vi "Get Public Events.vi"(8 "error in (no error)":errorcluster, 11 "LogEngine.lvclass":refnum<class "LogEngine.lvclass">) -> (0 "error out":errorcluster, 2 "PublicEvents":T1, 3 "LogEngine.lvclass":refnum<class "LogEngine.lvclass">)   [LabVIEW 2017, in "LogEngine.lvclass"]
doc: "Developed by Kevin Thompson\nkevin@thompsonengineering.net\n\nCopyright 2018-2020\nThompson Engineering, LLC"
uses:
  LogEngine.lvclass
  Data Types/TD LogEngine PublicEvents--cluster.ctl
  Ichor_Common/DataTypes/TD Async CmdMsg EventData--cluster.ctl
  Data Types/TD LoggerStateChanged EventData--cluster.ctl
  Data Types/TD Logger State Data--cluster.ctl
  Data Types/TD Logger State--enum.ctl
  LogEngine.lvclass/LogEngine.ctl
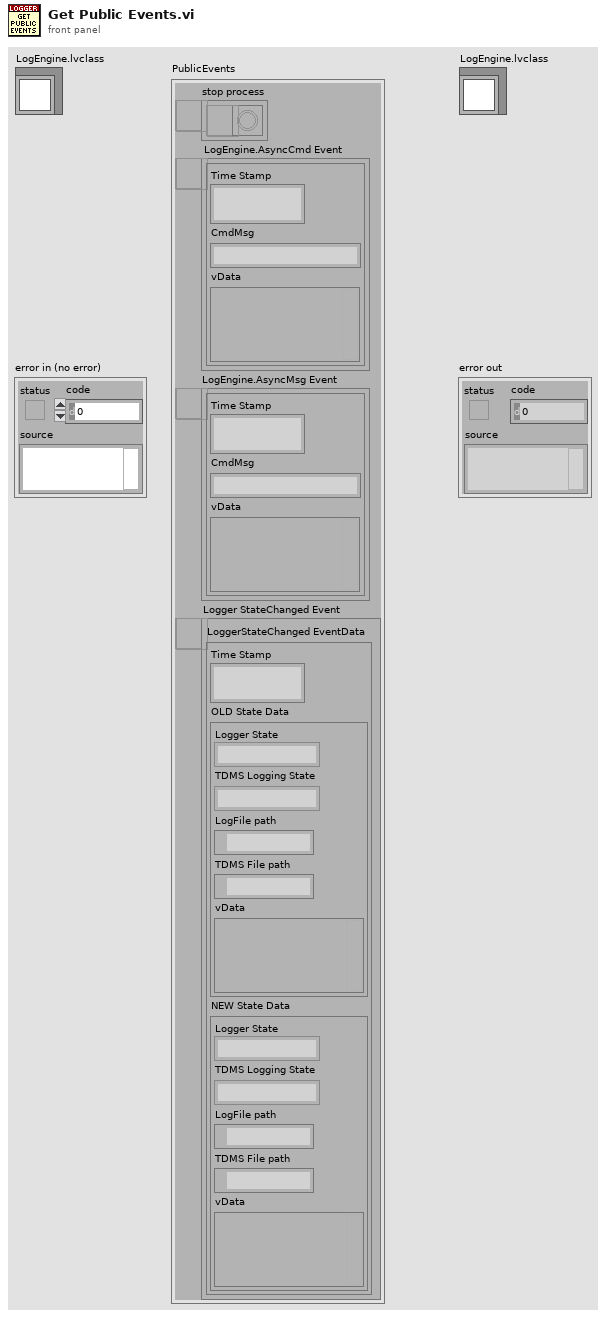
[diagram p1: front panel]
types:
  T1 = typedef "LogEngine.lvclass/TD LogEngine PublicEvents--cluster.ctl" = cluster{"stop process":refnum<user-event>, "LogEngine.AsyncCmd Event":refnum<user-event>, "LogEngine.AsyncMsg Event":refnum<user-event>, "Logger StateChanged Event":refnum<user-event>}
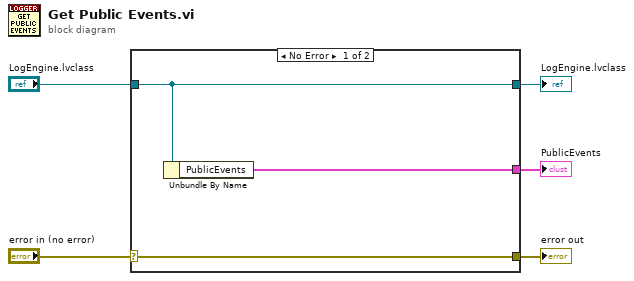
[diagram p0: block diagram]
diagram:
  n1 = case shown="No Error" "error in (no error)" {
    selector: "error in (no error)" -> [w8 w9]
    tunnel: [w8 w9] -> w4
    tunnel: [w7 w10] -> w2
    tunnel: "LogEngine.lvclass" -> [w7 w10]
    tunnel: [w6 _] -> w1
    frame No Error {
      n2 = Unbundle By Name(w7) -> ("PublicEvents"=w6:T1)
    }
    frame Error {
    }
  }
  "error out" <- w4
  "LogEngine.lvclass" <- w2
  "PublicEvents" <- w1
